vi "ShooterOverride.vi"(8 "Top Ball Sensor":bool, 9 "Collector Rear Speed":dbl, 10 "Throttle":dbl, 11 "Intake Speed":dbl) -> (2 "Intake Speed":dbl, 3 "Collecter Rear Speed":dbl)   [LabVIEW 2011]
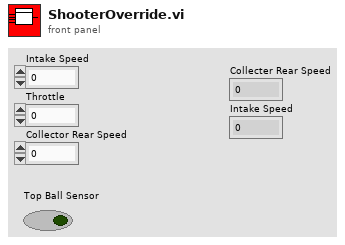
[diagram p1: front panel]
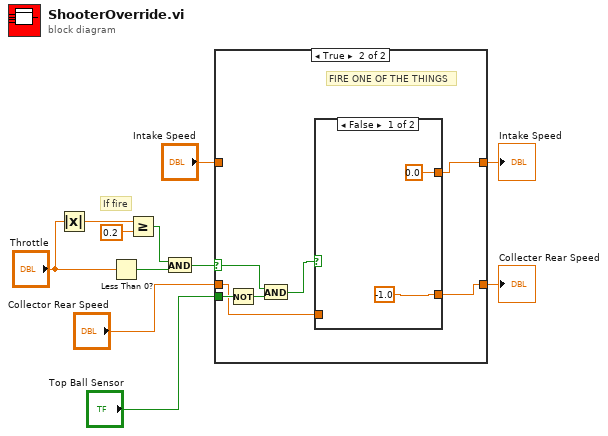
[diagram p0: block diagram]
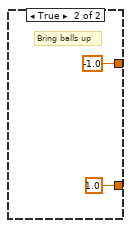
[diagram p3: hidden frame]
diagram:
  # "If fire"
  n1 = Absolute Value(x="Throttle") -> (abs(x)=w9:dbl)
  n2 = Less Than 0?(x="Throttle") -> (x < 0?=w8:bool)
  n3 = Greater Or Equal?(x=w9, y=0.2) -> (x >= y?=w11:bool)
  n4 = And(x=w11, y=w8) -> (x .and. y?=w6:bool)
  n5 = case shown="True" w6 {
    selector: w6 -> [_ w18]
    tunnel: [w12 w15] -> w5
    tunnel: [w13 w16] -> w4
    tunnel: "Intake Speed" -> [w13 _]
    tunnel: "Collector Rear Speed" -> [w12 w14]
    tunnel: "Top Ball Sensor" -> [_ w20]
    frame False {
    }
    frame True {
      # "FIRE ONE OF THE THINGS"
      n6 = Not(x=w20) -> (.not. x?=w19:bool)
      n7 = And(x=w18, y=w19) -> (x .and. y?=w17:bool)
      n8 = case shown="False" w17 {
        tunnel: [-1.0 1.0] -> w15
        tunnel: [0.0 -1.0] -> w16
        tunnel: w14 -> [_ _]
        frame False {
        }
        frame True {
          # "Bring balls up"
        }
      }
    }
  }
  "Collecter Rear Speed" <- w5
  "Intake Speed" <- w4
